vi "Call Records FGV.vi"(11 "Call Recorder Action":T1=enum."Read Values") -> (0 "Close-Detach calls":u32, 1 "Close-Close calls":u32, 2 "Initialize-Attach calls":u32, 3 "Initialize-Create calls":u32)   [LabVIEW 2020, in "MeasurementServerTests.lvlib" / "Fake Instrument.lvclass"]
uses:
  Fake Instrument.lvclass
  Call Recorder Action.ctl
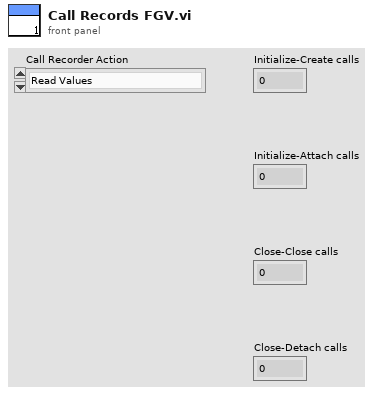
[diagram p1: front panel]
types:
  T1 = typedef "MeasurementServerTests.lvlib/Fake Instrument.lvclass/Call Recorder Action.ctl" = enum16{"Initialize", "Read Values", "Record Initialize-Create", "Record Initialize-Attach", "Record Close-Close", "Record Close-Detach"}
  T2 = cluster{"Initialize-Create calls":u32, "Initialize-Attach calls":u32, "Close-Close calls":u32, "Close-Detach calls":u32}
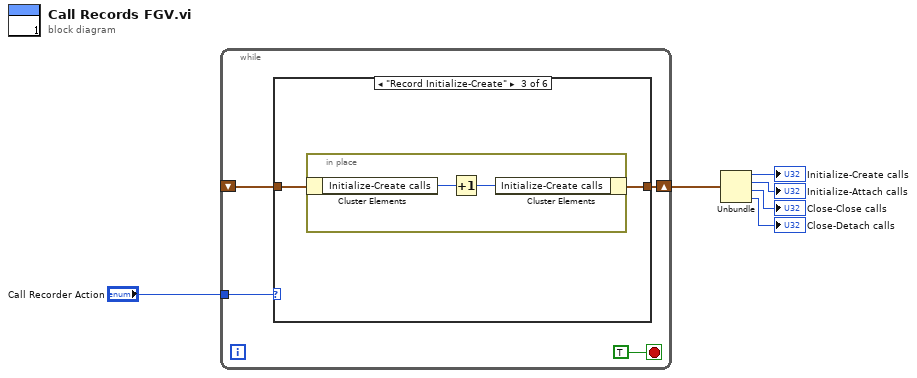
[diagram p0: block diagram]
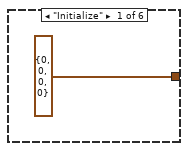
[diagram p2: hidden frame]
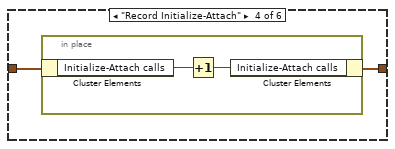
[diagram p4: hidden frame]
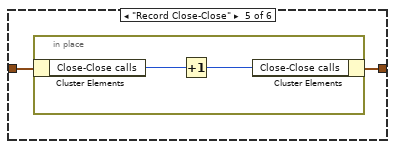
[diagram p5: hidden frame]
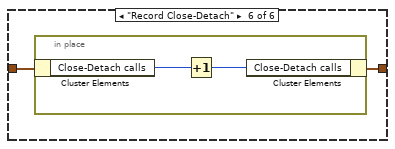
[diagram p6: hidden frame]
diagram:
  n1 = while {
    shift-right: [w9] -> w6
    shift-left: _ -> [w7]
    tunnel: "Call Recorder Action" -> [w8]
    stop <- TRUE stop-if-true
    n2 = case shown="\"Record Initialize-Create\"" w8 {
      tunnel: [T2 {"Initialize-Create calls"=0, "Initialize-Attach calls"=0, "Close-Close calls"=0, "Close-Detach calls"=0} ("Cluster") w12 w13 w17 w21 w25] -> w9
      tunnel: w7 -> [_ w12 w14 w18 w22 w26]
      frame "Initialize" {
      }
      frame "Read Values" {
      }
      frame "Record Initialize-Create" {
        n3 = in-place {
          n4 = in-place-cluster #1(w14) -> ("Initialize-Create calls"=w16:u32)
          n5 = Increment(x=w16) -> (x+1=w15:u32)
          n6 = in-place-cluster #1("Initialize-Create calls"=w15) -> (w13:T2)
        }
      }
      frame "Record Initialize-Attach" {
        n7 = in-place {
          n8 = in-place-cluster #2(w18) -> ("Initialize-Attach calls"=w20:u32)
          n9 = Increment(x=w20) -> (x+1=w19:u32)
          n10 = in-place-cluster #2("Initialize-Attach calls"=w19) -> (w17:T2)
        }
      }
      frame "Record Close-Close" {
        n11 = in-place {
          n12 = in-place-cluster #3(w22) -> ("Close-Close calls"=w24:u32)
          n13 = Increment(x=w24) -> (x+1=w23:u32)
          n14 = in-place-cluster #3("Close-Close calls"=w23) -> (w21:T2)
        }
      }
      frame "Record Close-Detach" {
        n15 = in-place {
          n16 = in-place-cluster #4(w26) -> ("Close-Detach calls"=w28:u32)
          n17 = Increment(x=w28) -> (x+1=w27:u32)
          n18 = in-place-cluster #4("Close-Detach calls"=w27) -> (w25:T2)
        }
      }
    }
  }
  n19 = Unbundle(w6) -> ("Initialize-Create calls"=→"Initialize-Create calls":u32, "Initialize-Attach calls"=→"Initialize-Attach calls":u32, "Close-Close calls"=→"Close-Close calls":u32, "Close-Detach calls"=→"Close-Detach calls":u32)
